vi "XimeaSettingsUpdate.vi"(8 "error in":errorcluster, 10 "Cluster":T1={"Harware Configuration"={"Camera"="cam1", "Frames Per Second"=15, "Simulate Recording"=TRUE, "Simulated Recording Sample"=path "", "Timestamp Method"=enum."System Timestamp"}, "Base Recording Path"=path "", "Type Of Recording"="", "Recording Codec"="", "TrackingSettings"={"Max Radius"=10, "Threshold"=122.53247, "ROI"={"Left"=1, "Top"=1, "Right"=2, "Bottom"=0, "Rotation"=0.0}}, "Calibration"={"Pixel Width (X)"=1.0, "Pixel Height (Y)"=1.0}, "Broadcast Length"=0} {"Broadcast Length" min=0; "TrackingSettings"."ROI"."Rotation" format="%.2f"; "TrackingSettings"."ROI"."Left" scale=0.0..1024.0; "TrackingSettings"."ROI"."Right" scale=0.0..1024.0; "TrackingSettings"."Threshold" scale=0.0..255.0}, 11 "Session In":T2="cam5") -> (0 "error out":errorcluster, 3 "IMAQdx Session":T2)   [LabVIEW 2017, in "ImageAcquisitionLibrary.lvlib"]
uses:
  ImageAcquisitionLibrary.lvlib
  <vilib>/userdefined/High Color/IMAQdx.ctl
  Settings.ctl
  Tracking/TrackingSettings.ctl
  Calibration.ctl
  <vilib>/Utility/error.llb/DialogType.ctl
  <resource>/objmgr/imaqdx.rc
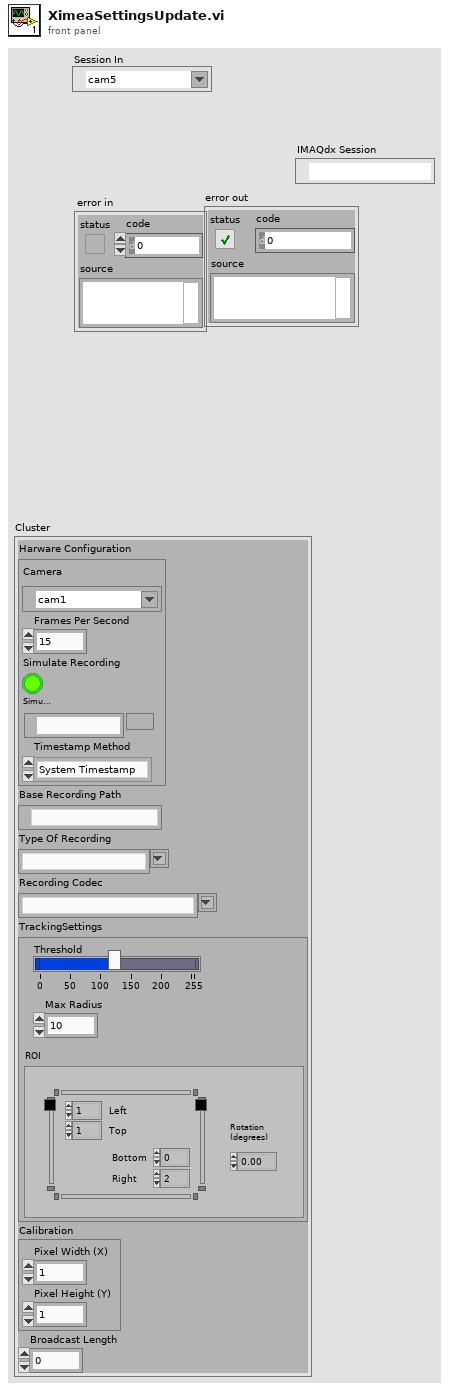
[diagram p1: front panel]
types:
  T1 = typedef "ImageAcquisitionLibrary.lvlib/Settings.ctl" = cluster{"Harware Configuration":cluster{"Camera":T2, "Frames Per Second":u32, "Simulate Recording":bool, "Simulated Recording Sample":path, "Timestamp Method":enum16{"System Timestamp", "Camera Timestamp", "IMAQdx Timestamp"}}, "Base Recording Path":path, "Type Of Recording":string, "Recording Codec":string, "TrackingSettings":T3, "Calibration":T5, "Broadcast Length":i32}
  T2 = typedef "IMAQdx.ctl" = refnum<k21>
  T3 = typedef "ImageAcquisitionLibrary.lvlib/TrackingSettings.ctl" = cluster{"Max Radius":i32, "Threshold":sgl, "ROI":T4}
  T4 = typedef "IMAQ Rectangle" = cluster{"Left":i32, "Top":i32, "Right":i32, "Bottom":i32, "Rotation":dbl}
  T5 = typedef "ImageAcquisitionLibrary.lvlib/Calibration.ctl" = cluster{"Pixel Width (X)":dbl, "Pixel Height (Y)":dbl}
  T6 = typedef "DialogType.ctl" = u16
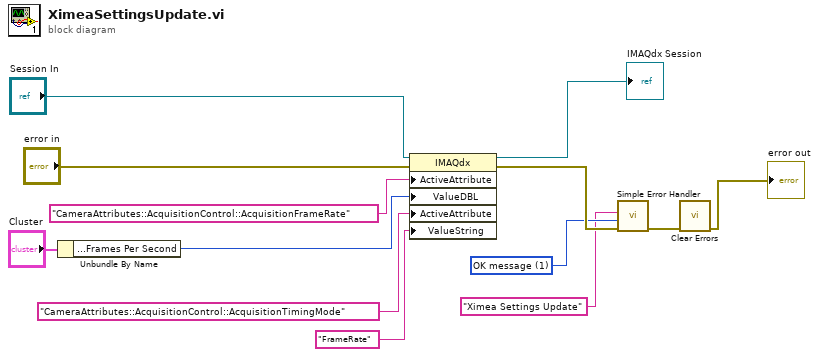
[diagram p0: block diagram]
diagram:
  w4 = T6 1 items=["no dialog", "OK message", "continue or stop message", "OK message + warnings", "continue/stop + warnings"] ("type of dialog (OK msg:1)")
  n1 = Unbundle By Name("Cluster") -> ("Harware Configuration.Frames Per Second"=w10:u32)
  n2 = property class="IMAQdx"(reference="Session In", error in="error in", "ActiveAttribute"="CameraAttributes::AcquisitionControl::AcquisitionFrameRate", "ValueDBL"=w10, "ActiveAttribute"="CameraAttributes::AcquisitionControl::AcquisitionTimingMode", "ValueString"="FrameRate" ("ActiveAttribute")) -> (reference out=→"IMAQdx Session":T2, error out=w5:errorcluster)
  n3 = call <vilib>:"Simple Error Handler.vi"("error source (\" \")"="Ximea Settings Update" ("error source (\" \")"), "type of dialog (OK msg:1)"=w4, "error in (no error)"=w5) -> ("error out"=w1:errorcluster)  [unwired: 2 in, 4 out]
  n4 = call <vilib>:"Clear Errors.vi"("error in (no error)"=w1) -> ("error out"=→"error out":errorcluster)  [unwired: 5 in, 1 out]
